vi "MakeFilepathString.vi"(1 "Project":string="Proj_VaporTubes\\Temp Dependence", 2 "Measurement number":i32=2, 3 "Extra":string="200C", 4 "Instrument":string="Lightfield") -> (5 "Date Folder":path=path "C:/Users/aspitarl/Git/MHDLab/Test Data/2018-06-28", 6 "Folder":path=path "C:/Users/aspitarl/Git/MHDLab/Test Data/2018-06-28/Proj_VaporTubes/Temp Dependence", 7 "Filename":string="Lightfield_200C_2.tdms")   [LabVIEW 2018]
uses:
  Global Variables.vi
panel:
  out "concatenated string":string="2018-06-28"
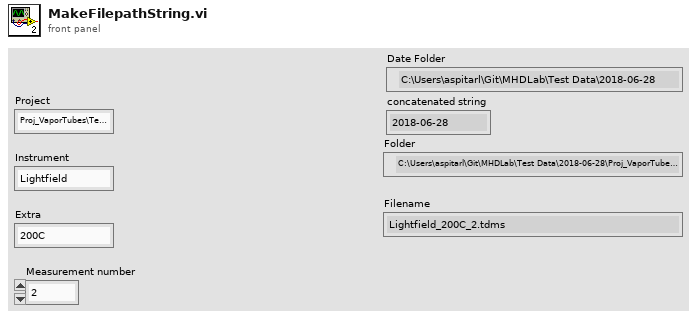
[diagram p1: front panel]
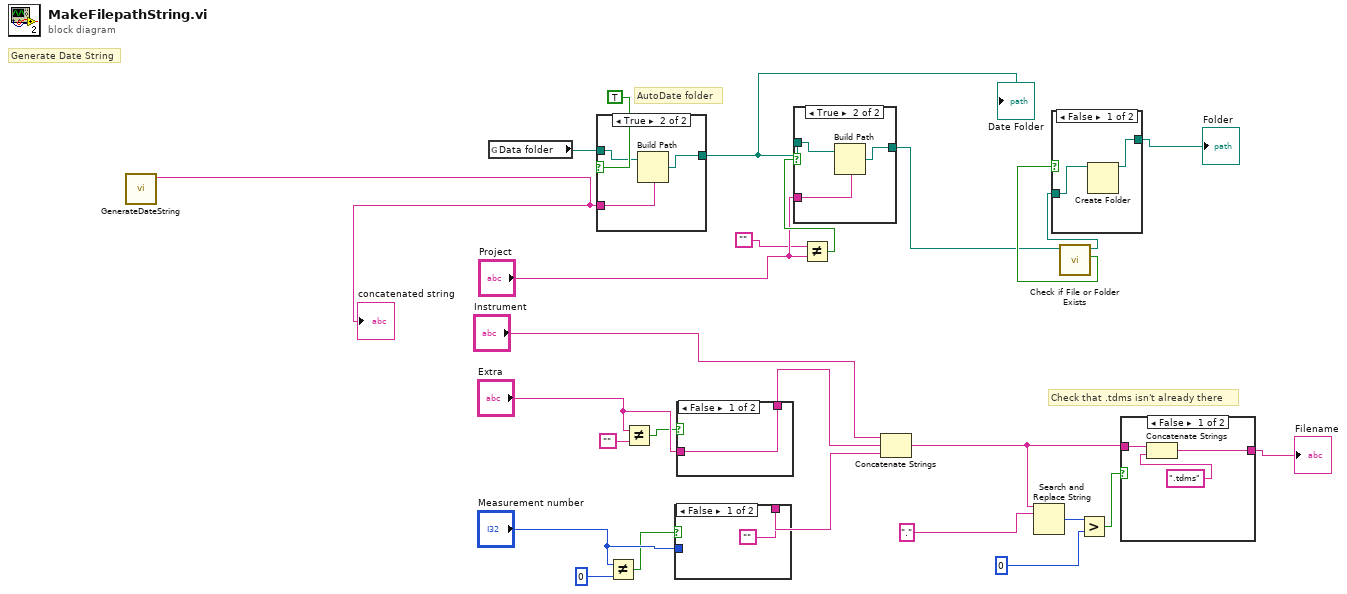
[diagram p0: block diagram]
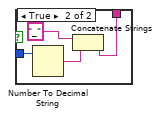
[diagram p2: hidden frame]
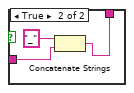
[diagram p3: hidden frame]
diagram:
  # "Generate Date String"
  # "Check that .tdms isn't already there"
  # "AutoDate folder"
  n1 = call "GenerateDateString.vi"() -> ("String"=w6:string)  [unwired: 11 in]
  "concatenated string" <- w6
  n2 = global read "Global Variables.vi" "Data folder"() -> (w1:path)
  n3 = case shown="True" TRUE ("Auto Date folder") {
    tunnel: w1 -> [w27 w30]
    tunnel: [w27 w28] -> w2
    tunnel: w6 -> [_ w29]
    frame False {
    }
    frame True {
      n4 = Build Path(base path=w30, name or relative path=w29) -> (appended path=w28:path)
    }
  }
  "Date Folder" <- w2
  n5 = Not Equal?(x="Measurement number", y=0) -> (x != y?=w21:bool)
  n6 = Not Equal?(x="Extra", y="") -> (x != y?=w18:bool)
  n7 = case shown="False" w21 {
    tunnel: ["" w34] -> w25
    tunnel: "Measurement number" -> [_ w33]
    frame False {
    }
    frame True {
      n8 = Number To Decimal String(number=w33) -> (decimal integer string=w32:string)  [unwired: 1 in]
      n9 = Concatenate Strings("_" ("element"), w32) -> (w34:string)
    }
  }
  n10 = case shown="False" w18 {
    tunnel: "Extra" -> [w36 w38]
    tunnel: [w36 w37] -> w24
    frame False {
    }
    frame True {
      n11 = Concatenate Strings("_" ("element"), w38) -> (w37:string)
    }
  }
  n12 = Not Equal?(x="", y="Project") -> (x != y?=w14:bool)
  n13 = case shown="True" w14 {
    tunnel: w2 -> [w40 w43]
    tunnel: [w40 w41] -> w3
    tunnel: "Project" -> [_ w42]
    frame False {
    }
    frame True {
      n14 = Build Path(base path=w43, name or relative path=w42) -> (appended path=w41:path)
    }
  }
  n15 = Concatenate Strings("Instrument", w24, w25) -> (w26:string)
  n16 = Search and Replace String(input string=w26, search string=".") -> (number of replacements=w9:i32)  [unwired: 6 in, 3 out]
  n17 = call <vilib>:"Check if File or Folder Exists.vi"("path"=w3) -> ("file or folder exists?"=w15:bool, "dup path"=w4:path)  [unwired: 8 in, 1 out]
  n18 = case shown="False" w15 {
    tunnel: w4 -> [w45 w46]
    tunnel: [w44 w46] -> w5
    frame False {
      n19 = Create Folder(path (use dialog)=w45) -> (created path=w44:path)  [unwired: 2 in, 2 out]
    }
    frame True {
    }
  }
  "Folder" <- w5
  n20 = Greater?(x=w9, y=0) -> (0:w11:bool)
  n21 = case shown="False" w11 {
    tunnel: [w48 w50] -> w16
    tunnel: w26 -> [w47 w50]
    frame False {
      n22 = Concatenate Strings(w47, ".tdms" ("string")) -> (w48:string)
    }
    frame True {
    }
  }
  "Filename" <- w16
